vi "Value_Combiner.vi"(4 "Precision (3)":string, 5 "String Array":string[](array[string])) -> (0 "Audit String":string, 1 "Output String":string)   [LabVIEW 2010]
uses:
  <vilib>/Analysis/NI_AALBase.lvlib
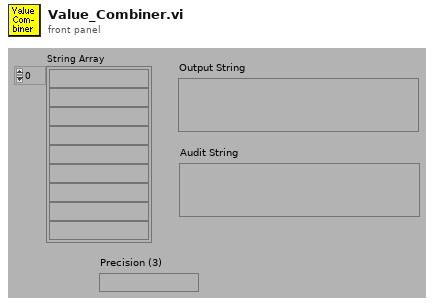
[diagram p1: front panel]
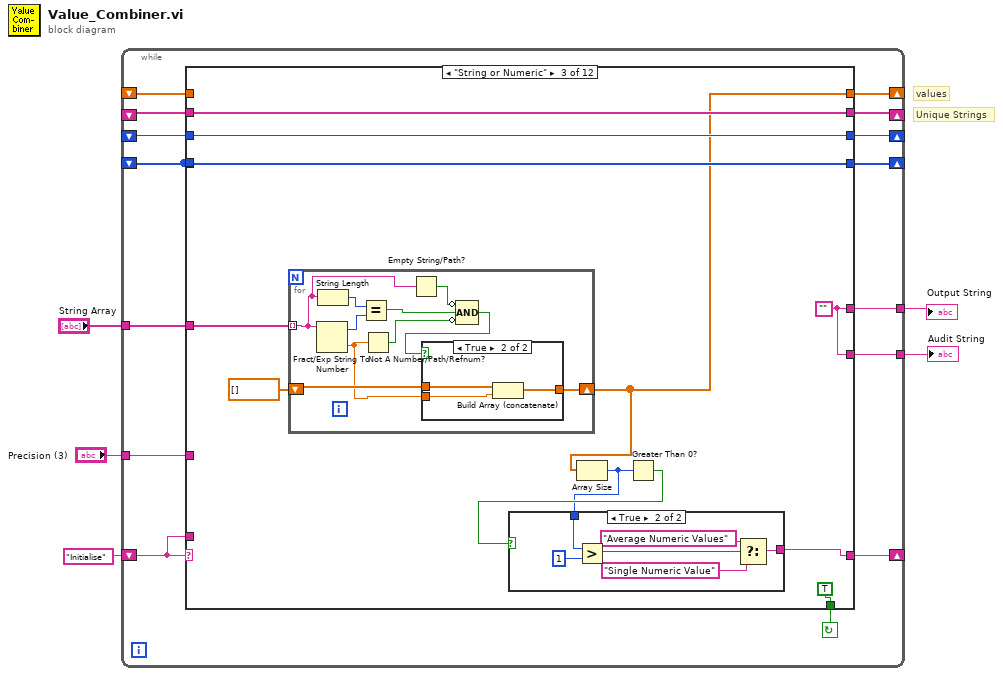
[diagram p0: block diagram]
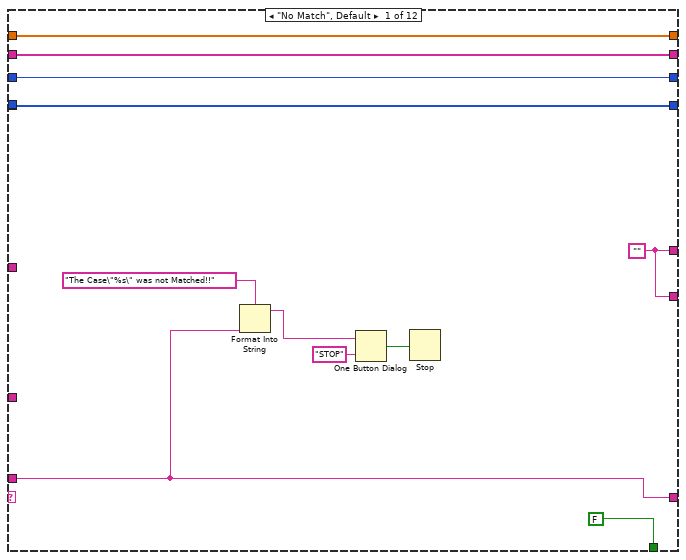
[diagram p2: hidden frame]
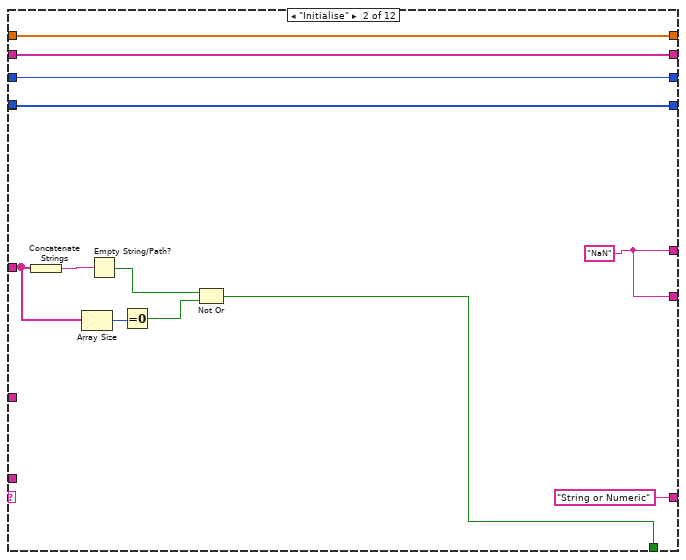
[diagram p3: hidden frame]
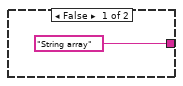
[diagram p4: hidden frame]
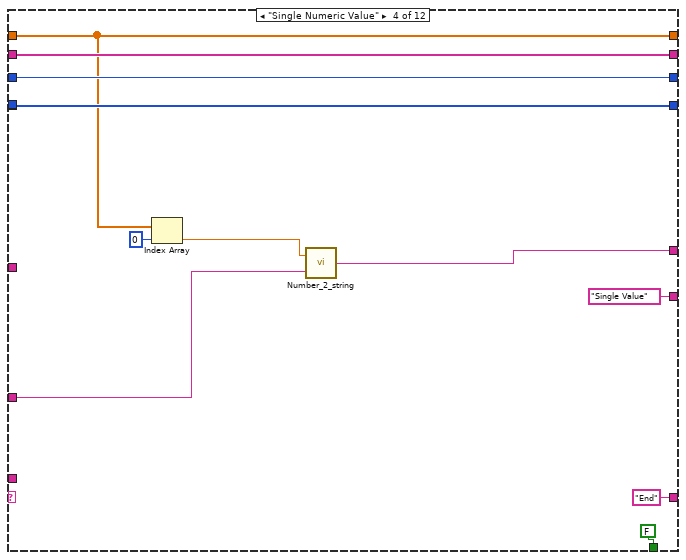
[diagram p6: hidden frame]
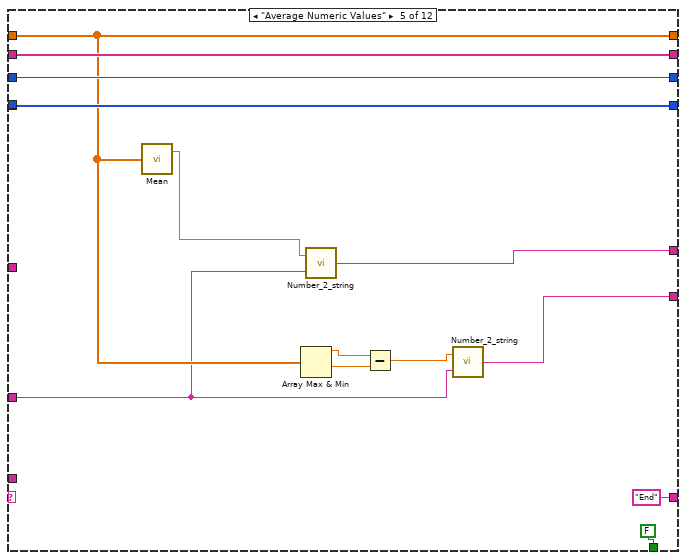
[diagram p7: hidden frame]
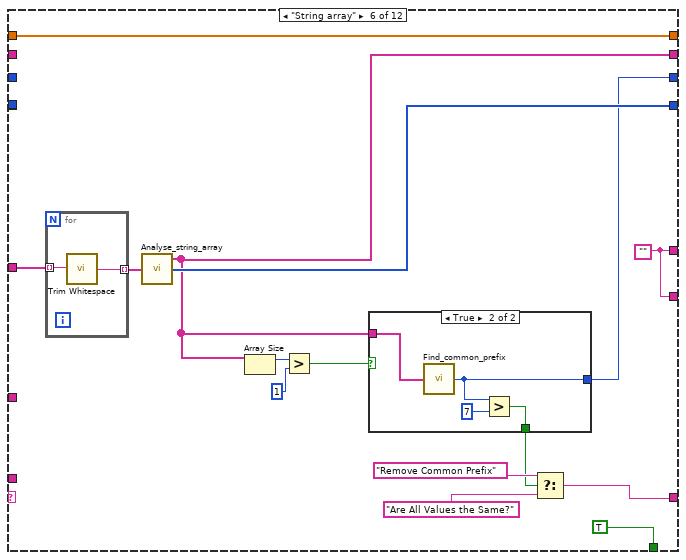
[diagram p8: hidden frame]
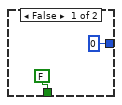
[diagram p9: hidden frame]
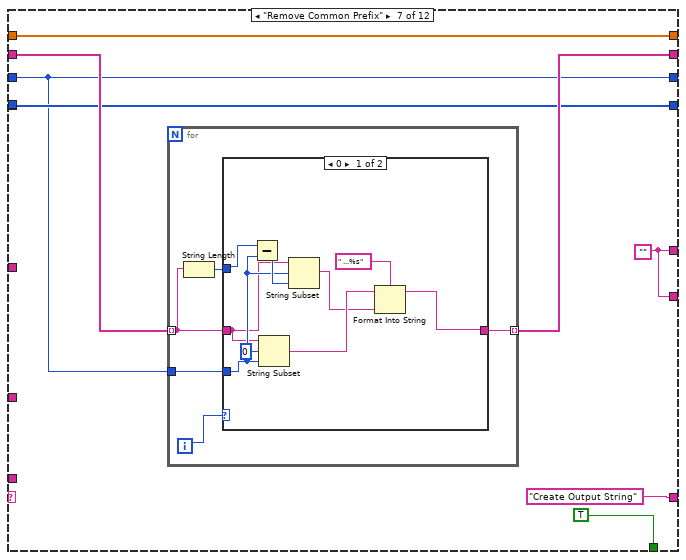
[diagram p10: hidden frame]
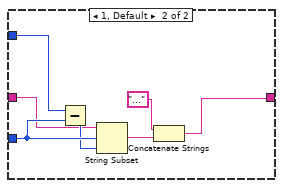
[diagram p11: hidden frame]
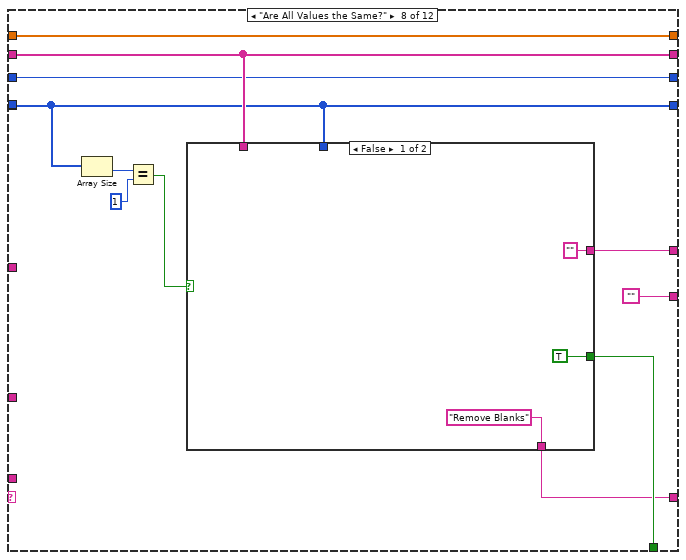
[diagram p12: hidden frame]
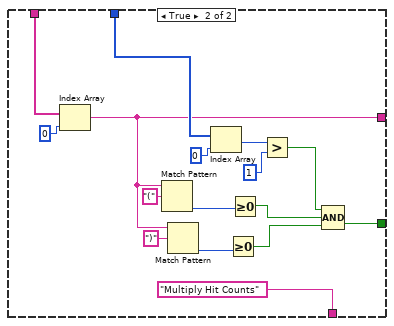
[diagram p13: hidden frame]
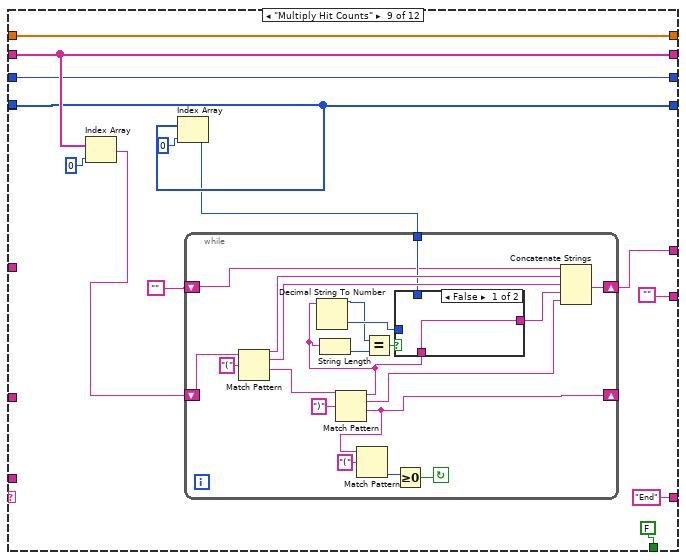
[diagram p14: hidden frame]
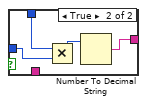
[diagram p15: hidden frame]
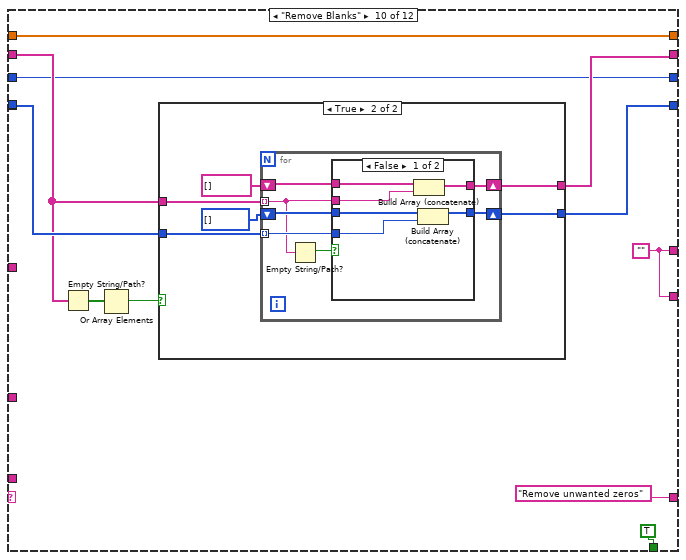
[diagram p16: hidden frame]
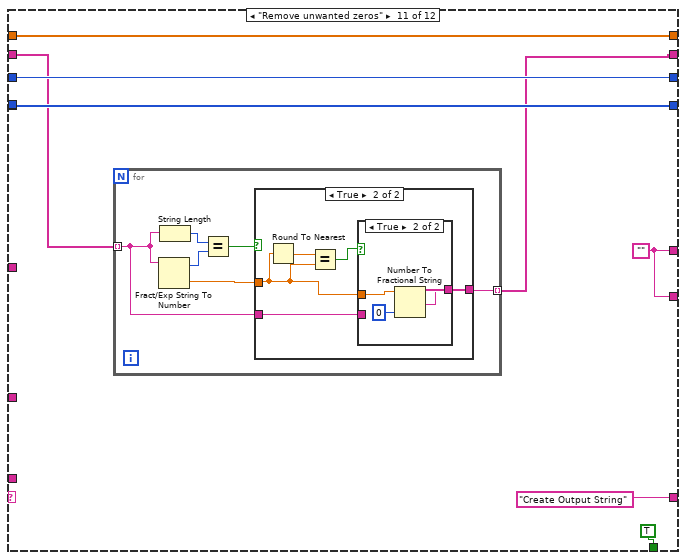
[diagram p19: hidden frame]
diagram:
  # "Unique Strings"
  # "values"
  n1 = while {
    shift-left: _ -> [w8]
    shift-right: [w9] -> _
    tunnel: [w10] -> w3
    shift-left: _ -> [w11]
    shift-right: [w12] -> _
    shift-left: _ -> [w13]
    shift-right: [w14] -> _
    shift-left: _ -> [w15]
    shift-right: [w19] -> _
    shift-left: "Initialise" -> [w16]
    shift-right: [w18] -> _
    tunnel: "String Array" -> [w20]
    tunnel: [w7] -> w2
    tunnel: "Precision (3)" -> [w6]
    stop <- w17 continue-if-true
    n2 = case shown="\"String or Numeric\"" w16 {
      tunnel: w20 -> [_ w38 w52 _ _ w106 _ _ _ _ _ _]
      tunnel: [w26 w43 w48 w82 w92 w113 w129 w162 w194 w226 w259 w294] -> w19
      tunnel: [w27 "String or Numeric" w46 "End" "End" w107 "Create Output String" w154 "End" "Remove unwanted zeros" "Create Output String" "Initialise"] -> w18
      tunnel: [FALSE w34 TRUE FALSE FALSE TRUE TRUE w156 FALSE TRUE TRUE FALSE] -> w17
      tunnel: w16 -> [w27 _ _ _ _ _ _ _ _ _ _ _]
      tunnel: w15 -> [w26 w43 _ w82 w92 w113 w129 w162 w194 w226 w259 w294]
      tunnel: [w24 w42 w53 w85 w98 w112 w125 w155 w191 w223 w258 w281] -> w14
      tunnel: w13 -> [w24 w42 w53 w85 w98 _ w125 w155 w191 w225 w258 w281]
      tunnel: w13 -> [_ _ _ _ _ _ _ _ _ _ _ _]
      tunnel: [w23 w41 w54 w86 w99 w102 w127 w159 w193 w224 w255 w290] -> w12
      tunnel: w11 -> [w23 w41 w54 w86 w99 _ w126 w159 w193 w222 w256 w290]
      tunnel: [w21 w32 w44 w78 w95 w100 w123 w153 w185 w220 w254 w284] -> w10
      tunnel: [w22 w33 w50 w83 w96 w111 w124 w158 w192 w221 w257 w283] -> w9
      tunnel: w8 -> [w22 w33 w50 w83 w96 _ w124 w158 w192 w221 w257 w283]
      tunnel: [w21 w32 w44 "Single Value" w87 w100 w123 "" "" w220 w254 ""] -> w7
      tunnel: w6 -> [_ _ _ w79 w88 _ _ _ _ _ _ _]
      frame "No Match", Default {
        w21 = ""
        n3 = Format Into String(format string="The Case\"%s\" was not Matched!!" ("Format String"), w27) -> (resulting string=w30:string)  [unwired: 2 in, 1 out]
        n4 = One Button Dialog(message=w30, button name ("OK")="STOP") -> (true=w25:bool)
        n5 = Stop(stop? (T)=w25) -> ()
      }
      frame "Initialise" {
        w32 = "NaN"
        n6 = Concatenate Strings(w38) -> (w39:string)
        n7 = Array Size(array=w38) -> (size(s)=w36:i32)
        n8 = Empty String/Path?(string/path=w39) -> (empty?=w37:bool)
        n9 = Equal To 0?(x=w36) -> (x = 0?=w35:bool)
        n10 = Not Or(1:w35, 2:w37) -> (0:w34:bool)
      }
      frame "String or Numeric" {
        w44 = ""
        n11 = for {
          tunnel: w52 -> [w68] mode=indexing
          shift-right: [w64] -> w48
          shift-left: dbl[] [] -> [w65]
          n12 = Fract/Exp String To Number(string=w68) -> (offset past number=w70:i32, number=w63:dbl)  [unwired: 3 out]
          n13 = String Length(string=w68) -> (length=w69:i32)
          n14 = Equal?(x=w69, y=w70) -> (x = y?=w67:bool)
          n15 = Not A Number/Path/Refnum?(number/path/refnum=w63) -> (NaN/Path/Refnum?=w62:bool)
          n16 = Empty String/Path?(string/path=w68) -> (empty?=w71:bool)
          n17 = Compound Arithmetic op=AND(invert w71, w67, invert w62) -> (w66:bool)
          n18 = case shown="True" w66 {
            tunnel: w65 -> [w72 w75]
            tunnel: w63 -> [_ w74]
            tunnel: [w72 w73] -> w64
            frame False {
            }
            frame True {
              n19 = Build Array (concatenate)(w75, w74) -> (w73:dbl[])
            }
          }
        }
        n20 = Array Size(array=w48) -> (size(s)=w45:i32)
        n21 = Greater Than 0?(x=w45) -> (x > 0?=w47:bool)
        n22 = case shown="True" w47 {
          tunnel: ["String array" w56] -> w46
          tunnel: w45 -> [_ w61]
          frame False {
          }
          frame True {
            n23 = Greater?(x=w61, y=1) -> (0:w59:bool)
            n24 = Select(t="Average Numeric Values", s=w59, f="Single Numeric Value") -> (s? t:f=w56:string)
          }
        }
      }
      frame "Single Numeric Value" {
        n25 = Index Array(array=w82, index=0) -> (element=w80:dbl)
        n26 = call "Number_2_string.vi"("precision"=w79, "number"=w80) -> ("String"=w78:string)
      }
      frame "Average Numeric Values" {
        n27 = call <vilib>:"Mean.vi"("X"=w92) -> ("mean"=w93:dbl)  [unwired: 1 out]
        n28 = Array Max & Min(array=w92) -> (max value=w91:dbl, min value=w90:dbl)  [unwired: 2 out]
        n29 = call "Number_2_string.vi"("precision"=w88, "number"=w93) -> ("String"=w95:string)
        n30 = Subtract(x=w91, y=w90) -> (x-y=w89:dbl)
        n31 = call "Number_2_string.vi"("precision"=w88, "number"=w89) -> ("String"=w87:string)
      }
      frame "String array" {
        w100 = ""
        n32 = for {
          tunnel: w106 -> [w116] mode=indexing
          tunnel: [w115] -> w105 mode=indexing
          n33 = call <vilib>:"Trim Whitespace.vi"("string"=w116) -> ("trimmed string"=w115:string)  [unwired: 1 in]
        }
        n34 = call "Analyse_string_array.vi"("String array"=w105) -> ("Unique strings"=w102:string[], "Frequency"=w112:i32[])  [unwired: 1 out]
        n35 = Array Size(array=w102) -> (size(s)=w104:i32)
        n36 = Greater?(x=w104, y=1) -> (0:w101:bool)
        n37 = case shown="True" w101 {
          tunnel: w102 -> [_ w122]
          tunnel: [0 ("Common Characters") w120] -> w111
          tunnel: [FALSE w119] -> w108
          frame False {
          }
          frame True {
            n38 = call "Find_common_prefix.vi"("Input Array"=w122) -> ("Common Characters"=w120:i32)
            n39 = Greater?(x=w120, y=7) -> (0:w119:bool)
          }
        }
        n40 = Select(t="Remove Common Prefix", s=w108, f="Are All Values the Same?") -> (s? t:f=w107:string)
      }
      frame "Remove Common Prefix" {
        w123 = ""
        n41 = for {
          tunnel: [w134] -> w127 mode=indexing
          tunnel: w126 -> [w132] mode=indexing
          tunnel: w124 -> [w133]
          i -> [w135]
          n42 = String Length(string=w132) -> (length=w131:i32)
          n43 = case shown="0" w135 {
            tunnel: [w136 w148] -> w134
            tunnel: w132 -> [w140 w149]
            tunnel: w133 -> [w141 w151]
            tunnel: w131 -> [w142 w145]
            frame 0 {
              n44 = Subtract(x=w142, y=w141) -> (x-y=w143:i32)
              n45 = String Subset(string=w140, offset (0)=0, length (rest)=w141) -> (substring=w139:string)
              n46 = String Subset(string=w140, offset (0)=w141, length (rest)=w143) -> (substring=w138:string)
              n47 = Format Into String(format string=" ...%s" ("Format String"), initial string=w139, w138) -> (resulting string=w136:string)  [unwired: 1 in, 1 out]
            }
            frame 1, Default {
              n48 = Subtract(x=w145, y=w151) -> (x-y=w150:i32)
              n49 = String Subset(string=w149, offset (0)=w151, length (rest)=w150) -> (substring=w147:string)
              n50 = Concatenate Strings("..." ("Substring"), w147) -> (w148:string)
            }
          }
        }
      }
      frame "Are All Values the Same?" {
        n51 = Array Size(array=w155) -> (size(s)=w160:i32)
        n52 = Equal?(x=w160, y=1) -> (x = y?=w157:bool)
        n53 = case shown="False" w157 {
          tunnel: w159 -> [_ w180]
          tunnel: ["" ("f") w166] -> w153
          tunnel: [TRUE w173] -> w156
          tunnel: w155 -> [_ w171]
          tunnel: ["Remove Blanks" "Multiply Hit Counts"] -> w154
          frame False {
          }
          frame True {
            n54 = Index Array(array=w180, index=0 ("Index")) -> (element=w166:string)
            n55 = Match Pattern(string=w166, regular expression="(") -> (offset past match=w177:i32)  [unwired: 4 out]
            n56 = Match Pattern(string=w166, regular expression=")") -> (offset past match=w176:i32)  [unwired: 4 out]
            n57 = Index Array(array=w171, index=0 ("Index")) -> (element=w170:i32)
            n58 = Greater Or Equal To 0?(x=w176) -> (x >= 0?=w175:bool)
            n59 = Greater Or Equal To 0?(x=w177) -> (x >= 0?=w174:bool)
            n60 = Greater?(x=w170, y=1) -> (0:w168:bool)
            n61 = Compound Arithmetic op=AND(w168, w174, w175) -> (w173:bool)
          }
        }
      }
      frame "Multiply Hit Counts" {
        n62 = Index Array(array=w193, index=0 ("Index")) -> (element=w188:string)
        n63 = Index Array(array=w191, index=0 ("Index")) -> (element=w187:i32)
        n64 = while {
          shift-right: [w209] -> _
          shift-left: w188 -> [w211]
          shift-right: [w200] -> w185
          shift-left: "" -> [w199]
          tunnel: w187 -> [w203]
          stop <- w207 continue-if-true
          n65 = Match Pattern(string=w211, regular expression="(") -> (before substring=w206:string, match substring=w205:string, after substring=w212:string)  [unwired: 2 out]
          n66 = Match Pattern(string=w212, regular expression=")") -> (before substring=w195:string, match substring=w201:string, after substring=w209:string)  [unwired: 2 out]
          n67 = Decimal String To Number(string=w195) -> (offset past number=w197:i32, number=w204:i32)  [unwired: 2 out]
          n68 = String Length(string=w195) -> (length=w198:i32)
          n69 = Match Pattern(string=w209, regular expression="(") -> (offset past match=w208:i32)  [unwired: 4 out]
          n70 = Equal?(x=w197, y=w198) -> (x = y?=w196:bool)
          n71 = case shown="False" w196 {
            tunnel: w204 -> [_ w219]
            tunnel: w203 -> [_ w218]
            tunnel: [w215 w216] -> w202
            tunnel: w195 -> [w215 _]
            frame False {
            }
            frame True {
              n72 = Multiply(x=w218, y=w219) -> (x*y=w217:i32)
              n73 = Number To Decimal String(number=w217) -> (decimal integer string=w216:string)  [unwired: 1 out]
            }
          }
          n74 = Greater Or Equal To 0?(x=w208) -> (x >= 0?=w207:bool)
          n75 = Concatenate Strings(w199, w206, w205, w202, w201) -> (w200:string)
        }
      }
      frame "Remove Blanks" {
        w220 = ""
        n76 = Empty String/Path?(string/path=w222) -> (empty?=w228:bool[])
        n77 = Or Array Elements(Boolean array=w228) -> (logical OR=w227:bool)
        n78 = case shown="True" w227 {
          tunnel: w222 -> [w231 w233]
          tunnel: w225 -> [w232 w238]
          tunnel: [w231 w235] -> w224
          tunnel: [w232 w234] -> w223
          frame False {
          }
          frame True {
            n79 = for {
              shift-right: [w242] -> w235
              shift-left: string[] [] -> [w243]
              shift-right: [w241] -> w234
              shift-left: i32[] [] -> [w244]
              tunnel: w233 -> [w239] mode=indexing
              tunnel: w238 -> [w240] mode=indexing
              n80 = Empty String/Path?(string/path=w239) -> (empty?=w245:bool)
              n81 = case shown="False" w245 {
                tunnel: w244 -> [w251 w252]
                tunnel: w243 -> [w250 w253]
                tunnel: [w249 w253] -> w242
                tunnel: [w248 w252] -> w241
                tunnel: w239 -> [w247 _]
                tunnel: w240 -> [w246 _]
                frame False {
                  n82 = Build Array (concatenate)(w250, w247) -> (w249:string[])
                  n83 = Build Array (concatenate)(w251, w246) -> (w248:i32[])
                }
                frame True {
                }
              }
            }
          }
        }
      }
      frame "Remove unwanted zeros" {
        w254 = ""
        n84 = for {
          tunnel: w256 -> [w262] mode=indexing
          tunnel: [w263] -> w255 mode=indexing
          n85 = Fract/Exp String To Number(string=w262) -> (offset past number=w267:i32, number=w264:dbl)  [unwired: 3 out]
          n86 = String Length(string=w262) -> (length=w266:i32)
          n87 = Equal?(x=w266, y=w267) -> (x = y?=w265:bool)
          n88 = case shown="True" w265 {
            tunnel: w264 -> [_ w271]
            tunnel: [w268 w270] -> w263
            tunnel: w262 -> [w268 w269]
            frame False {
            }
            frame True {
              n89 = Round To Nearest(number=w271) -> (nearest integer value=w273:dbl)
              n90 = Equal?(x=w273, y=w271) -> (x = y?=w272:bool)
              n91 = case shown="True" w272 {
                tunnel: w271 -> [_ w277]
                tunnel: [w274 w276] -> w270
                tunnel: w269 -> [w274 _]
                frame False {
                }
                frame True {
                  n92 = Number To Fractional String(number=w277, precision (6)=i16 0) -> (F-format string=w276:string)  [unwired: 2 out]
                }
              }
            }
          }
        }
      }
      frame "Create Output String" {
        n93 = Equal?(x=w281, y=1) -> (x = y?=w280:bool[])
        n94 = And Array Elements(Boolean array=w280) -> (logical AND=w279:bool)
        n95 = for {
          shift-right: [w298] -> w288
          shift-left: "" -> [w299]
          tunnel: w290 -> [w297] mode=indexing
          tunnel: w281 -> [w296] mode=indexing
          tunnel: w279 -> [w295]
          n96 = case shown="True" w295 {
            tunnel: w299 -> [w304 w308]
            tunnel: [w303 w307] -> w298
            tunnel: w297 -> [w302 w306]
            tunnel: w296 -> [w301 _]
            frame False {
              n97 = Format Into String(format string="%s (%d);  " ("Format String"), initial string=w304, w302, w301) -> (resulting string=w303:string)  [unwired: 1 in, 1 out]
            }
            frame True {
              n98 = Format Into String(format string="%s;  " ("Format String"), initial string=w308, w306) -> (resulting string=w307:string)  [unwired: 1 in, 1 out]
            }
          }
        }
        n99 = String Length(string=w288) -> (length=w286:i32)
        n100 = Subtract(x=w286, y=2) -> (x-y=w285:i32)
        n101 = String Subset(string=w288, offset (0)=0, length (rest)=w285) -> (substring=w284:string)
      }
    }
  }
  "Output String" <- w3
  "Audit String" <- w2
